vi "XML config file parser.vi"(2 "Tag Name":string, 3 "XML File Path":path) -> (0 "Out":string, 1 "In":string)   [LabVIEW 2009]
uses:
  <vilib>/xml/NI_XML.lvlib
  <libdir>/resource/objmgr/DOMUserDefRef.rc
  <vilib>/xml/Close Reference(Node).vi
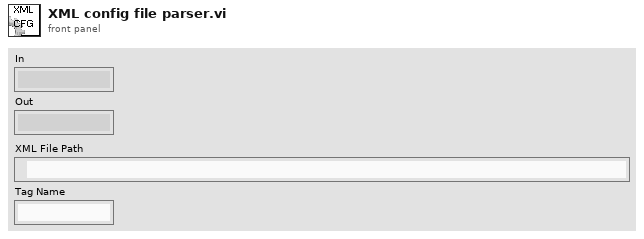
[diagram p1: front panel]
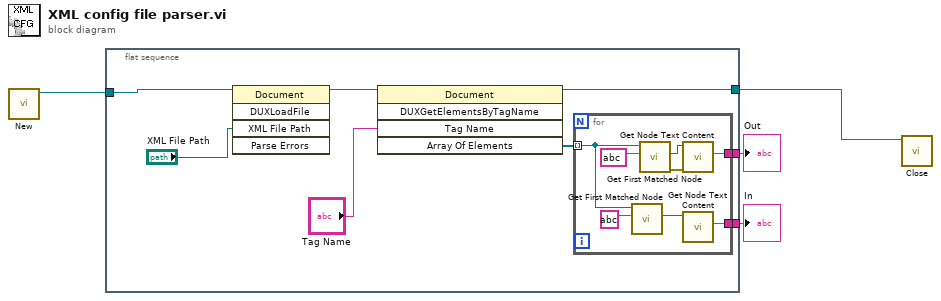
[diagram p0: block diagram]
diagram:
  n1 = call <vilib>:"New.vi"() -> ("DOM document out"=w4:refnum<k20>)  [unwired: 8 in, 1 out]
  n2 = flat-sequence {
    tunnel: w4 -> [w12]
    tunnel: [w7] -> w3
    tunnel: [w6] -> w2
    tunnel: [w5] -> w1
    frame #0 {
      n3 = invoke class="Document" method="DUXLoadFile"(reference=w12, "XML File Path"="XML File Path") -> (reference out=w8:refnum<k20>)  [unwired: 3 in, 4 out]
      n4 = invoke class="Document" method="DUXGetElementsByTagName"(reference=w8, "Tag Name"="Tag Name") -> (reference out=w5:refnum<k20>, "Array Of Elements"=w9:refnum<k20>[])  [unwired: 3 in, 3 out]
      n5 = for {
        tunnel: [w19] -> w7
        tunnel: [w16] -> w6
        tunnel: w9 -> [w13] mode=indexing
        n6 = call <vilib>:"Get First Matched Node.vi"("XPath expression"=string ? ("Tag Name"), "node in"=w13) -> ("node result"=w15:refnum<k20>)  [unwired: 7 in, 2 out]
        n7 = call <vilib>:"Get First Matched Node.vi"("XPath expression"=string ? ("Tag Name"), "node in"=w13) -> ("error out"=w18:errorcluster, "node result"=w14:refnum<k20>)  [unwired: 7 in, 1 out]
        n8 = call <vilib>:"Get Node Text Content.vi"("error in (no error)"=w18, "node in"=w14) -> ("node text"=w16:string)  [unwired: 7 in, 2 out]
        n9 = call <vilib>:"Get Node Text Content.vi"("node in"=w15) -> ("node text"=w19:string)  [unwired: 8 in, 2 out]
      }
    }
  }
  n10 = call-poly <vilib>:"Close.vi"("node"=w1) -> ()  [unwired: 8 in, 1 out]
  "In" <- w3
  "Out" <- w2
